vi "Actor Core.vi"(8 "error in":errorcluster, 11 "SpectrumAnalyzerUI in":refnum<class "SpectrumAnalyzerUI.lvclass">) -> (0 "error out":errorcluster, 3 "Actor out":refnum<class "Actor.lvclass">)   [LabVIEW 2023, in "SpectrumAnalyzerUI.lvlib" / "SpectrumAnalyzerUI.lvclass"]
doc: "(<B>Filename</B>: Actor Framework.lvlib:Actor.lvclass:Actor Core.vi)\n\nReceives messages to the actor, reacts to them, and initiates any error handling that may shut the actor down.\n\nDescendant classes may override this VI to append parallel tasks for the actor to complete while it handles messages. Overrides use the Call Parent Class Method node."
uses:
  SpectrumAnalyzerUI.lvclass
  <vilib>/ActorFramework/Actor/Actor.lvclass
  <vilib>/ActorFramework/Message Enqueuer/Message Enqueuer.lvclass
  Measurement_Type.ctl
  ConcreteClasses/ConcreteInstrumentClasses/KeysightN9020B/KeysightN9020B.lvclass
  <vilib>/ActorFramework/Actor/Actor.lvclass/Actor.ctl
  <vilib>/ActorFramework/Message Enqueuer/Message Enqueuer.lvclass/Message Enqueuer.ctl
  SpectrumAnalyzerUI.lvclass/SpectrumAnalyzerUI.ctl
  Interfaces/AbstractInstrumentClasses/SpectrumAnalyzer_LV/SpectrumAnalyzer Messages/ConfigureSpectrum Msg/ConfigureSpectrum Msg.lvclass/ConfigureSpectrum Msg.ctl
  Interfaces/AbstractInstrumentClasses/SpectrumAnalyzer_LV/SpectrumAnalyzer Messages/SetAverages Msg/SetAverages Msg.lvclass/SetAverages Msg.ctl
  Interfaces/InitDeinitInterface/InitDeinit Messages/Init Msg/Init Msg.lvclass/Init Msg.ctl
  Interfaces/AbstractInstrumentClasses/SpectrumAnalyzer_LV/SpectrumAnalyzer Messages/SetTrigger Msg/SetTrigger Msg.lvclass/SetTrigger Msg.ctl
  Interfaces/AbstractInstrumentClasses/SpectrumAnalyzer_LV/SpectrumAnalyzer Messages/SetAmplitudeRange Msg/SetAmplitudeRange Msg.lvclass/SetAmplitudeRange Msg.ctl
  <vilib>/ActorFramework/Message Enqueuer/Init from Existing Queue.vi
  <vilib>/ActorFramework/Message Enqueuer/Enqueue.vi
  Interfaces/AbstractInstrumentClasses/SpectrumAnalyzer_LV/SpectrumAnalyzer Messages/GetSpectrum Msg/GetSpectrum Msg.lvclass
  Interfaces/AbstractInstrumentClasses/SpectrumAnalyzer_LV/SpectrumAnalyzer Messages/ConfigureSpectrum Msg/ConfigureSpectrum Msg.lvclass
  Interfaces/AbstractInstrumentClasses/SpectrumAnalyzer_LV/SpectrumAnalyzer Messages/SetAverages Msg/SetAverages Msg.lvclass
  Interfaces/InitDeinitInterface/InitDeinit Messages/DeInit Msg/DeInit Msg.lvclass
  Interfaces/InitDeinitInterface/InitDeinit Messages/Init Msg/Init Msg.lvclass
  Interfaces/AbstractInstrumentClasses/SpectrumAnalyzer_LV/SpectrumAnalyzer Messages/SetTrigger Msg/SetTrigger Msg.lvclass
  Interfaces/AbstractInstrumentClasses/SpectrumAnalyzer_LV/SpectrumAnalyzer Messages/SetAmplitudeRange Msg/SetAmplitudeRange Msg.lvclass
  <vilib>/ActorFramework/Stop Msg/Stop Msg.lvclass
  <vilib>/ActorFramework/Message Priority Queue/Priority Enqueue.vi
  ConcreteClasses/ConcreteInstrumentClasses/KeysightN9020B/KeysightN9020B.lvlib
panel:
  out "output cluster":cluster{"Frequency":dbl[], "Amplitude":dbl[]}(graph)
  out "S-Meas Norm":dbl[][](graph)
  out "N-Meas":dbl[][](graph)
  out "S-Meas":dbl[][](graph)
  out "E-Meas":dbl[][](graph)
  out "appended array":dbl[][](graph)
  out "Measuring":bool=TRUE
  in  "attenuation":dbl caption="attenuation (dB)" min=0.0 max=10.0 step=0.1
  in  "reference level offset":dbl
  in  "reference level":dbl
  in  "Resolution BW":dbl=520.0 caption="Resolution BW (MHz)"
  in  "center frequency":dbl=520.0 caption="Center Frequency (MHz)"
  in  "span":dbl=1000.0 caption="Frequency span (MHz)"
  in  "Base Name":string="test"
  in  "file (use dialog)":path=path "D:/test"
  in  "S measurement":bool
  in  "N measurement":bool
  in  "E measurement":bool
  in  "Source":i32(ring)=1 items=["External"=1, "Immediate"=2, "Software"=3, "AC Line"=4, "Video"=5]
  in  "Trigger On":bool
  in  "ExternalTriggerLevel":dbl=1.0 caption="Trigger Level"
  out "Exiting":bool=TRUE
  out "Connected":bool
  in  "Connect":bool
  out "Measurement Type":T1=enum."S-Meas"
  out "N9020B Enqueuer":refnum<class "Message Enqueuer.lvclass">
  in  "VISA resource name":refnum<visa-resource-name>
  in  "instrument handle":refnum<k15>="N9020B"
  in  "Averages":i32
  in  "Show Spectrum":bool
  out "Self Enqueuer":refnum<class "Message Enqueuer.lvclass">
  in  "Stop Button":bool
  in  "Normalization":enum32{"(S-N)/(N-E)", "(S-E)/(E)"}(radio)=enum."(S-E)/(E)"
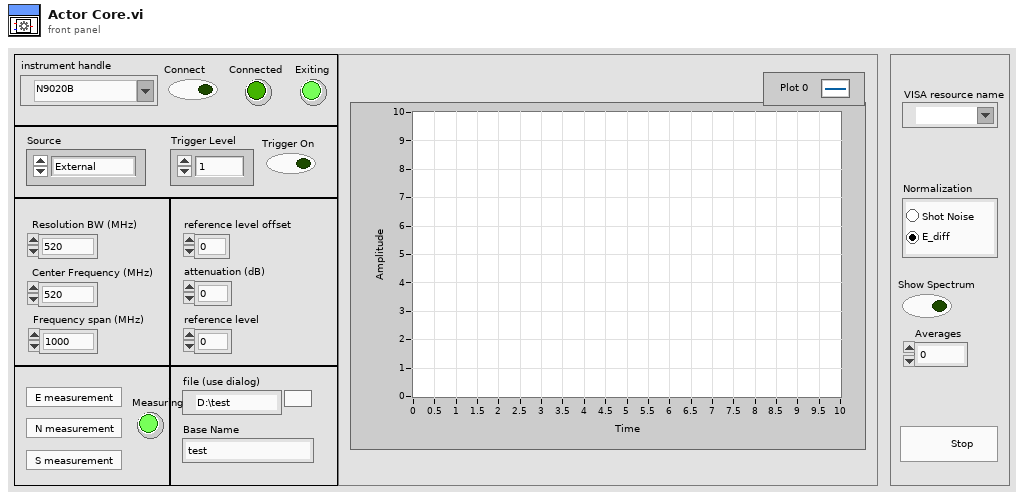
[diagram p1: front panel]
types:
  T1 = typedef "KeysightN9020B.lvlib/Measurement_Type.ctl" = enum16{"N-Meas", "S-Meas", "E-Meas", "Av_S vs Power"}
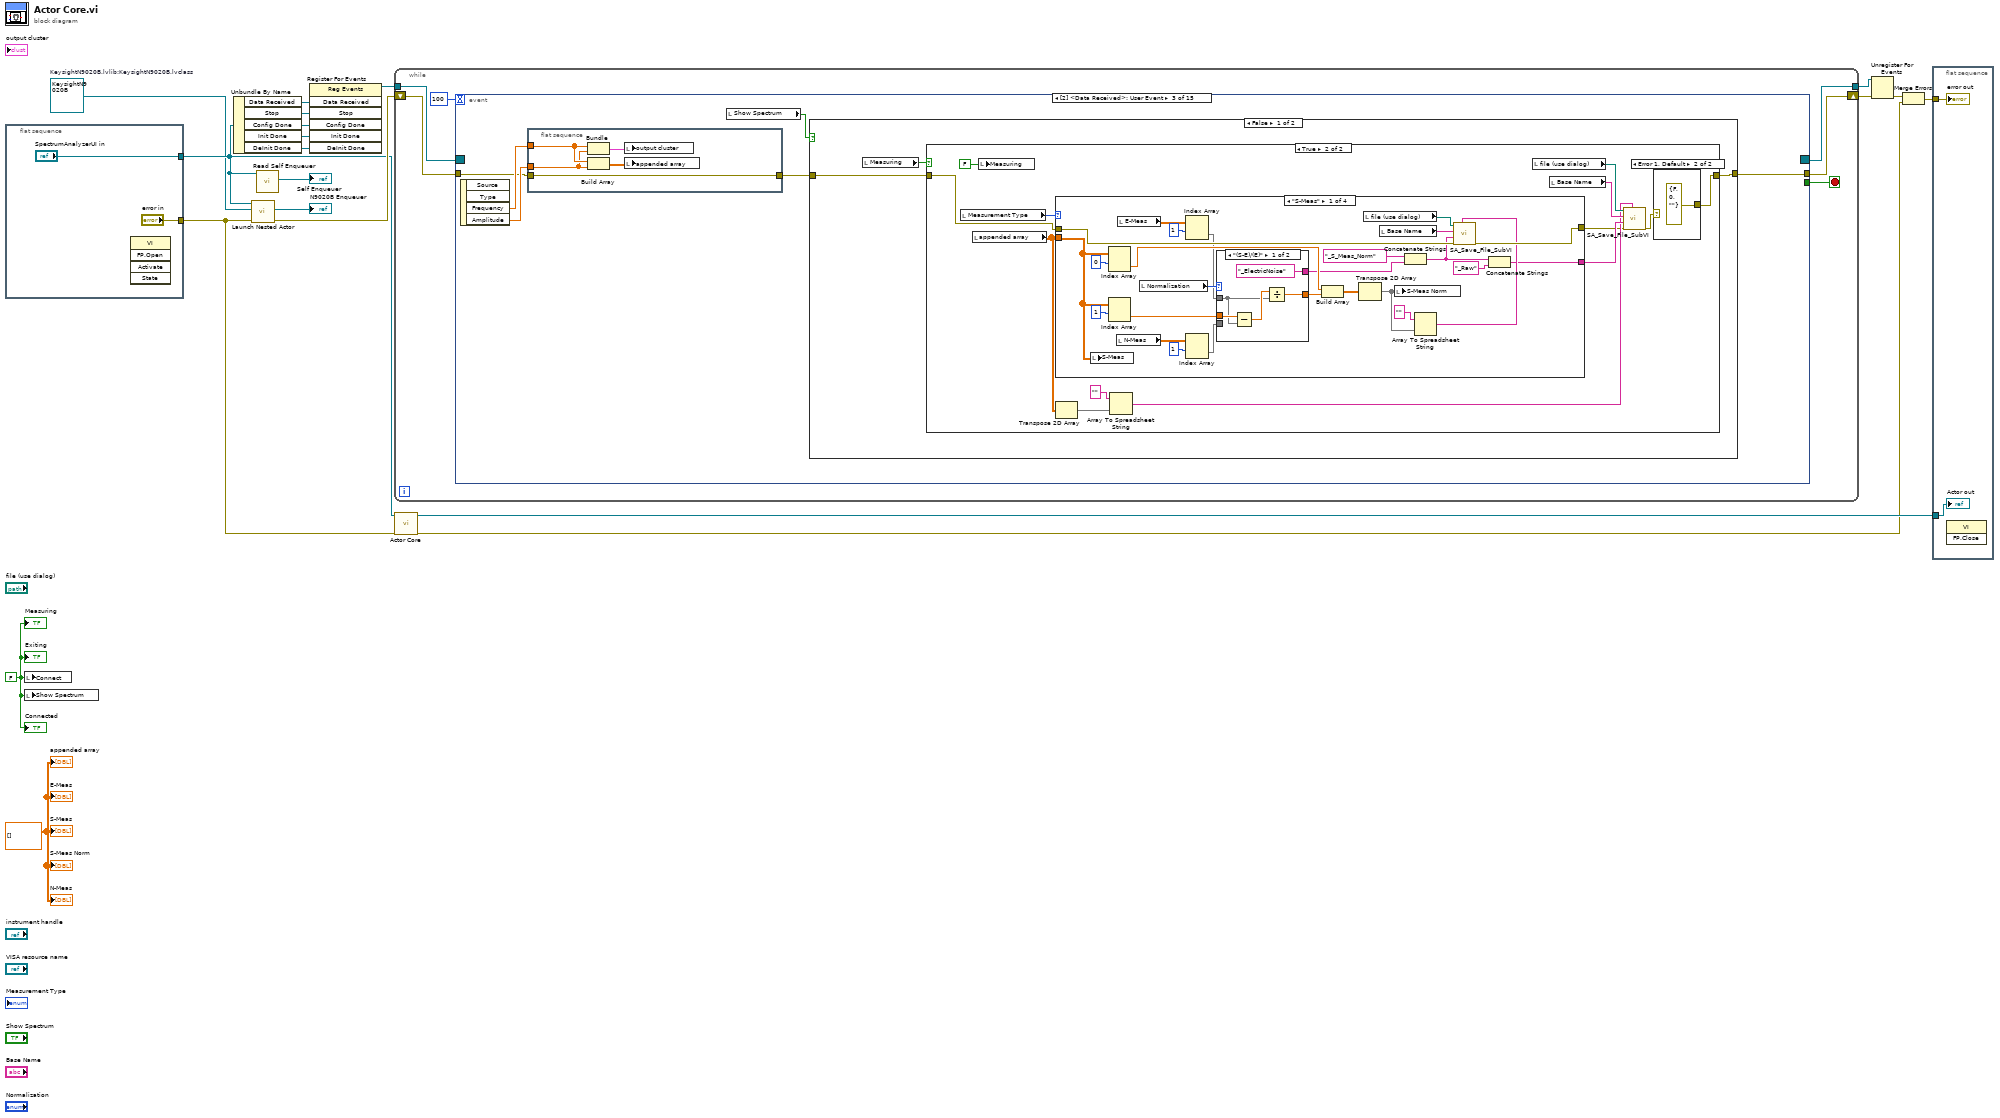
[diagram p0: block diagram]
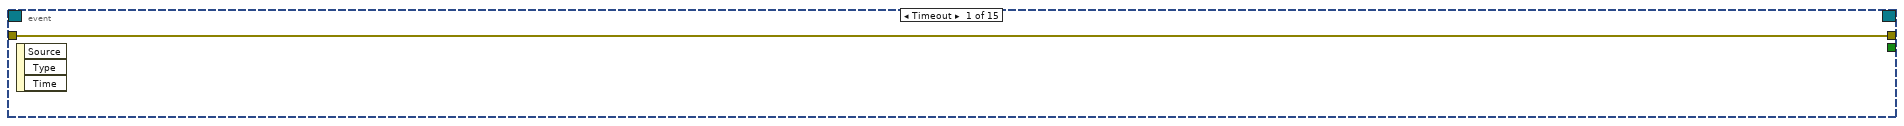
[diagram p2: hidden frame]
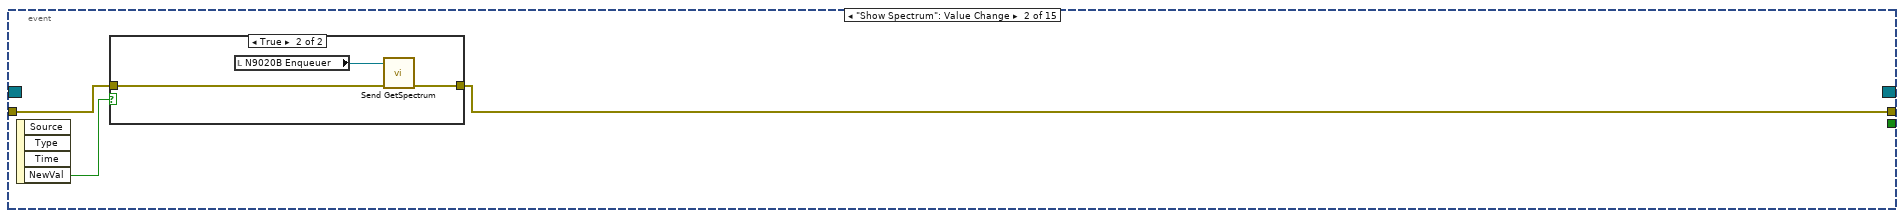
[diagram p3: hidden frame]
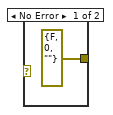
[diagram p6: hidden frame]
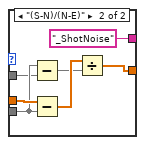
[diagram p7: hidden frame]
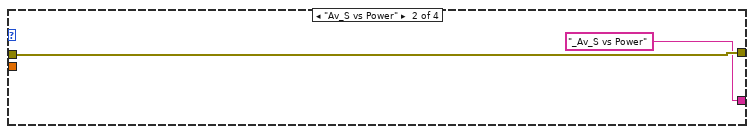
[diagram p8: hidden frame]
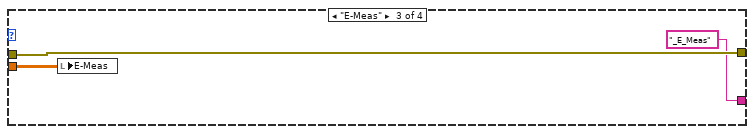
[diagram p9: hidden frame]
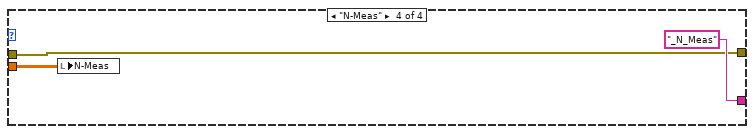
[diagram p10: hidden frame]
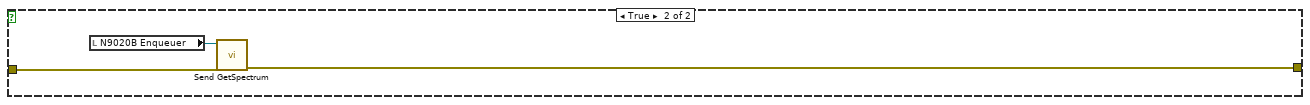
[diagram p11: hidden frame]
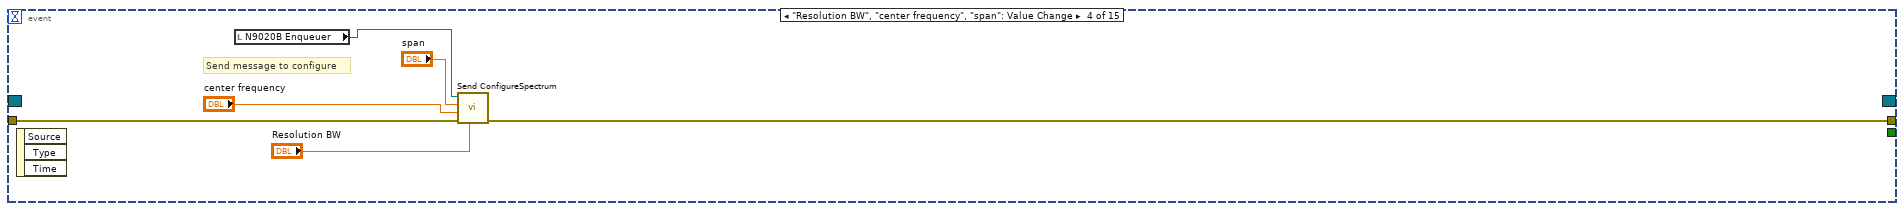
[diagram p12: hidden frame]
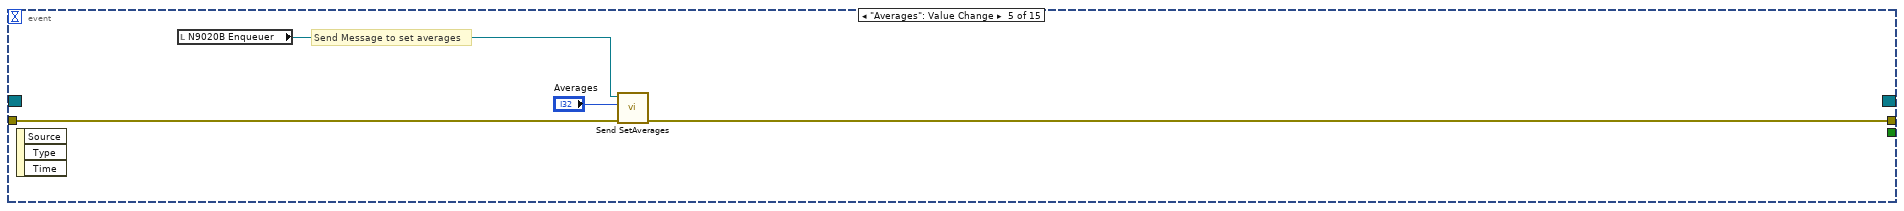
[diagram p13: hidden frame]
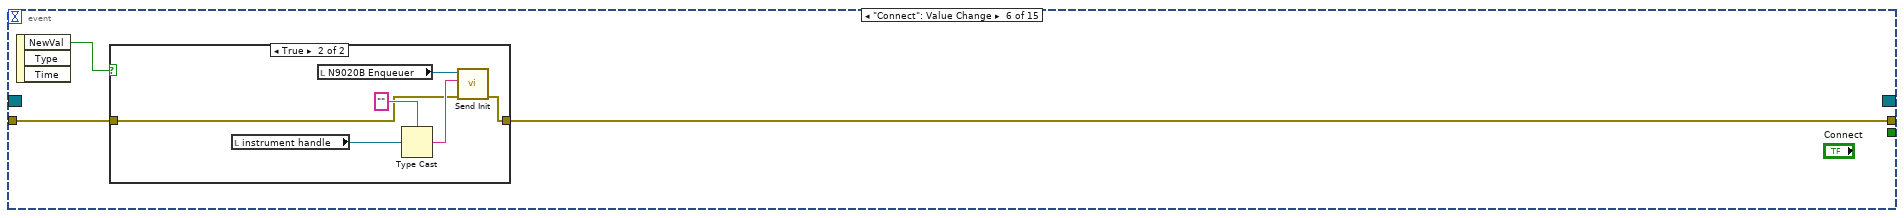
[diagram p14: hidden frame]
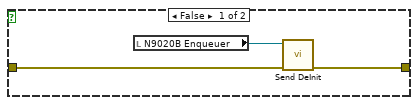
[diagram p15: hidden frame]
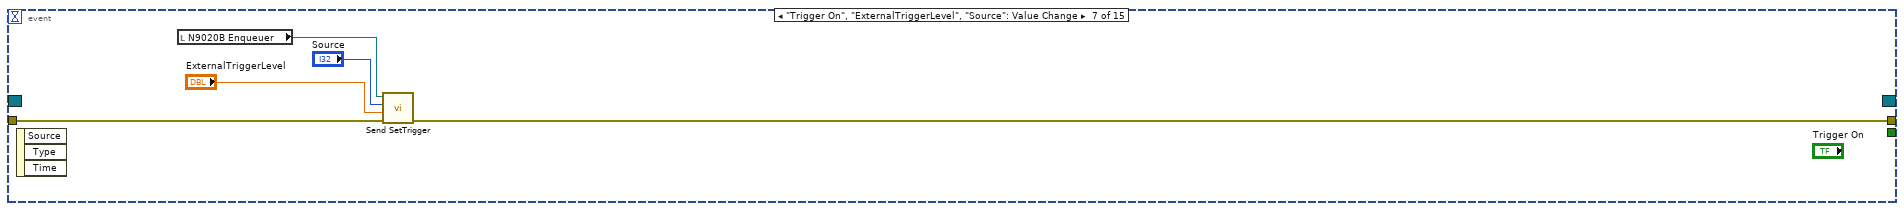
[diagram p16: hidden frame]
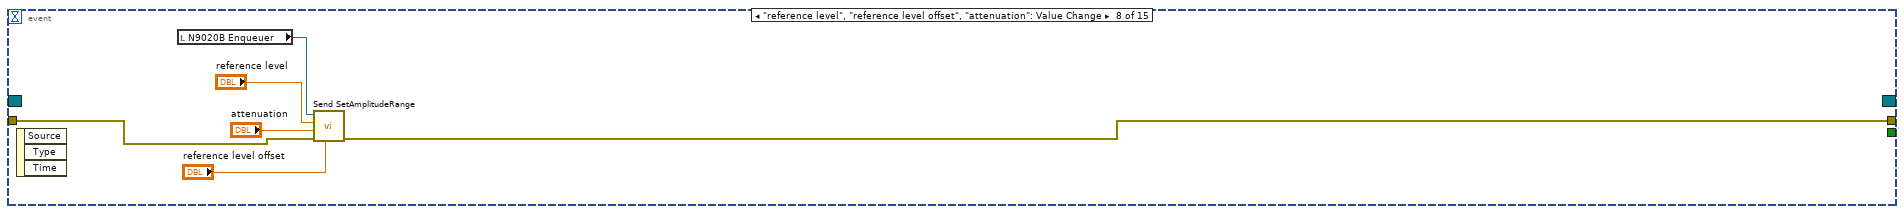
[diagram p17: hidden frame]
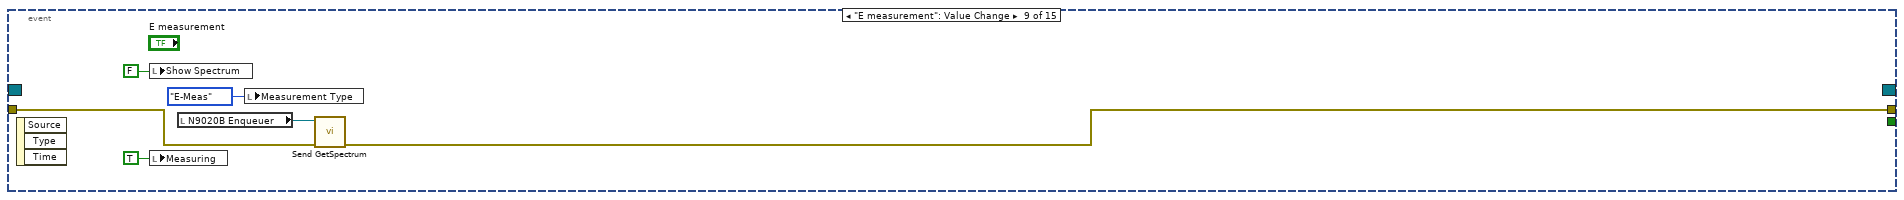
[diagram p18: hidden frame]
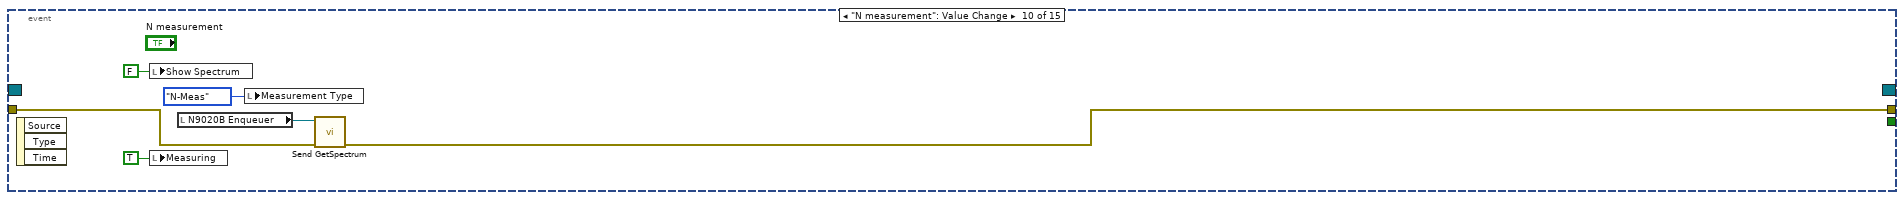
[diagram p19: hidden frame]
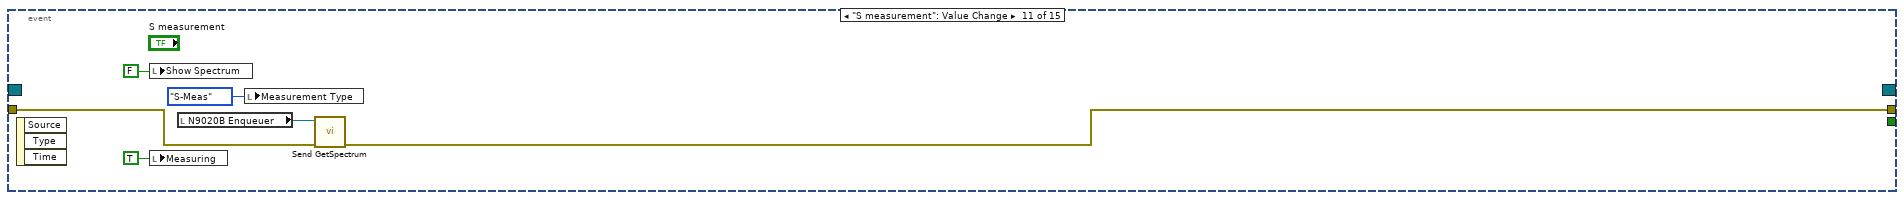
[diagram p20: hidden frame]
diagram:
  w1 = dbl[][] [] ("appended array")
  w3 = refnum<class "KeysightN9020B.lvclass"> refnum  # KeysightN9020B.lvlib:KeysightN9020B.lvclass
  w2 = FALSE ("Connected")
  n1 = flat-sequence {
    tunnel: ["error in"] -> w18
    tunnel: ["SpectrumAnalyzerUI in"] -> w15
    frame #0 {
      n2 = invoke class="VI" method="FP.Open"() -> ()  [unwired: 5 in, 5 out]
    }
  }
  n3 = local write "Connect"(w2) -> ()
  n4 = local write "Show Spectrum"(w2) -> ()
  n5 = Unbundle By Name(w15) -> ("Data Received"=w14:refnum<user-event>, "Stop"=w13:refnum<user-event>, "Config Done"=w12:refnum<user-event>, "Init Done"=w11:refnum<user-event>, "DeInit Done"=w9:refnum<user-event>)
  n6 = call <vilib>:"Launch Nested Actor.vi"("error in (no error)"=w18, "Nested Actor"=w3, "Caller Actor in"=w15) -> ("error out"=w16:errorcluster, "Nested Actor's Enqueuer"=→"N9020B Enqueuer":refnum<class "Message Enqueuer.lvclass">)  [unwired: 6 in, 1 out]
  n7 = call <vilib>:"Read Self Enqueuer.vi"("Actor"=w15) -> ("Self Enqueuer"=→"Self Enqueuer":refnum<class "Message Enqueuer.lvclass">)  [unwired: 10 in]
  n8 = register-events(w14, w13, w12, w11, w9) -> (reference out=w10:refnum<event-registration>)  [unwired: 2 in, 1 out]
  n9 = while {
    shift-right: [w27] -> w8
    shift-left: w16 -> [w28]
    tunnel: w10 -> [w25]
    tunnel: [w23] -> w4
    stop <- w24 stop-if-true
    n10 = event shown="[2] <Data Received>: User Event" {
      selector: w25 -> [_ _ _ _ _ _ _ _ _ _ _ _ _ _ _]
      dyn-events: [_ _ _ _ _ _ _ _ _ _ _ _ _ _ _] -> w23
      timeout: 100 -> [_ _ _ _ _ _ _ _ _ _ _ _ _ _ _]
      tunnel: w28 -> [w29 w31 w38 w117 w123 w128 w140 w147 w152 w158 w162 w170 w178 w182 w190]
      tunnel: [w29 w32 w41 w116 w122 w127 w139 w146 w151 w157 w161 w169 w178 w181 w190] -> w27
      tunnel: [_ _ _ _ _ _ _ _ _ _ _ _ _ _ TRUE] -> w24
      event Timeout {
        n11 = event-data() -> ()  [unwired: 1 in, 3 out]
      }
      event "Show Spectrum": Value Change {
        n12 = event-data() -> ("NewVal"=w30:bool)  [unwired: 1 in, 3 out]
        n13 = case shown="True" w30 {
          tunnel: w31 -> [w33 w35]
          tunnel: [w33 w34] -> w32
          frame False {
          }
          frame True {
            n14 = local read "N9020B Enqueuer"() -> (w36:refnum<class "Message Enqueuer.lvclass">)
            n15 = call "Send GetSpectrum.vi"("error in (no error)"=w35, "Message Enqueuer"=w36) -> ("error out"=w34:errorcluster)  [unwired: 8 in, 1 out]
          }
        }
      }
      event User Event {
        n16 = event-data() -> ("Frequency"=w40:dbl[], "Amplitude"=w39:dbl[])  [unwired: 1 in, 2 out]
        n17 = flat-sequence {
          tunnel: w40 -> [w45]
          tunnel: w39 -> [w44]
          tunnel: [w47] -> w37
          tunnel: w38 -> [w47]
          frame #0 {
            n18 = Bundle("Frequency"=w45, "Amplitude"=w44) -> (w46:cluster{"Frequency":dbl[], "Amplitude":dbl[]})  [unwired: 1 in]
            n19 = Build Array(w45, w44) -> (w43:dbl[][])
            n20 = local write "output cluster"(w46) -> ()
            n21 = local write "appended array"(w43) -> ()
          }
        }
        n22 = local read "Show Spectrum"() -> (w42:bool)
        n23 = case shown="False" w42 {
          tunnel: w37 -> [w48 w114]
          tunnel: [w49 w113] -> w41
          frame False {
            n24 = local read "Measuring"() -> (w50:bool)
            n25 = case shown="True" w50 {
              tunnel: [w51 w53] -> w49
              tunnel: w48 -> [w51 w63]
              frame False {
              }
              frame True {
                n26 = local read "Measurement Type"() -> (w64:T1)
                n27 = local read "appended array"() -> (w56:dbl[][])
                n28 = local write "Measuring"(FALSE ("Measuring")) -> ()
                n29 = case shown="\"S-Meas\"" w64 {
                  tunnel: [w88 w106 w109 w111] -> w52
                  tunnel: w63 -> [w89 w106 w109 w111]
                  tunnel: [w67 "_Av_S vs Power" ("string") "_E_Meas" ("string") "_N_Meas" ("string")] -> w59
                  tunnel: w56 -> [w79 _ w107 w110]
                  frame "S-Meas" {
                    n30 = local write "S-Meas"(w79) -> ()
                    n31 = Index Array(array=w79, index (row)=0) -> (element=w78:dbl[])  [unwired: 1 in]
                    n32 = Index Array(array=w79, index (row)=1) -> (element=w81:dbl[])  [unwired: 1 in]
                    n33 = local read "N-Meas"() -> (w83:dbl[][])
                    n34 = local read "E-Meas"() -> (w73:dbl[][])
                    n35 = local read "Normalization"() -> (w92:enum32{"(S-N)/(N-E)", "(S-E)/(E)"})
                    n36 = Index Array(array=w73, index (row)=1) -> (element=w72:dbl[])  [unwired: 1 in]
                    n37 = Index Array(array=w83, index (row)=1) -> (element=w82:dbl[])  [unwired: 1 in]
                    n38 = case shown="\"(S-E)/(E)\"" w92 {
                      tunnel: w72 -> [w95 w99]
                      tunnel: w81 -> [w97 w104]
                      tunnel: [w94 w102] -> w77
                      tunnel: w82 -> [_ w100]
                      tunnel: ["_ElectricNoise" ("string") "_ShotNoise" ("string")] -> w70
                      frame "(S-E)/(E)" {
                        n39 = Subtract(x=w97, y=w95) -> (x-y=w96:dbl[])
                        n40 = Divide(x=w96, y=w95) -> (x/y=w94:dbl[])
                      }
                      frame "(S-N)/(N-E)" {
                        n41 = Subtract(x=w100, y=w99) -> (x-y=w101:dbl[])
                        n42 = Subtract(x=w104, y=w100) -> (x-y=w103:dbl[])
                        n43 = Divide(x=w103, y=w101) -> (x/y=w102:dbl[])
                      }
                    }
                    n44 = Build Array(w78, w77) -> (w76:dbl[][])
                    n45 = Transpose 2D Array(2D array=w76) -> (transposed array=w75:dbl[][])
                    n46 = local read "file (use dialog)"() -> (w91:path)
                    n47 = local read "Base Name"() -> (w90:string)
                    n48 = local write "S-Meas Norm"(w75) -> ()
                    n49 = Concatenate Strings("_S_Meas_Norm" ("string"), w70) -> (w69:string)
                    n50 = Array To Spreadsheet String(array=w75, 3:"" ("format string")) -> (spreadsheet string=w86:string)  [unwired: 1 in]
                    n51 = call "SA_Save_File_SubVI.vi"("spreadsheet string"=w86, "error in (no error)"=w89, "string"=w69, "Base Name"=w90, "file (use dialog)"=w91) -> ("error out"=w88:errorcluster)  [unwired: 6 in]
                    n52 = Concatenate Strings(w69, "_Raw" ("string")) -> (w67:string)
                  }
                  frame "Av_S vs Power" {
                  }
                  frame "E-Meas" {
                    n53 = local write "E-Meas"(w107) -> ()
                  }
                  frame "N-Meas" {
                    n54 = local write "N-Meas"(w110) -> ()
                  }
                }
                n55 = Transpose 2D Array(2D array=w56) -> (transposed array=w55:dbl[][])
                n56 = Array To Spreadsheet String(array=w55, 3:"" ("format string")) -> (spreadsheet string=w58:string)  [unwired: 1 in]
                n57 = local read "file (use dialog)"() -> (w61:path)
                n58 = local read "Base Name"() -> (w60:string)
                n59 = call "SA_Save_File_SubVI.vi"("spreadsheet string"=w58, "error in (no error)"=w52, "string"=w59, "Base Name"=w60, "file (use dialog)"=w61) -> ("error out"=w54:errorcluster)  [unwired: 6 in]
                n60 = case shown="Error 1, Default" w54 {
                  tunnel: [errorcluster {"status"=FALSE, "code"=0, "source"=""} ("error out") errorcluster {"status"=FALSE, "code"=0, "source"=""} ("error out")] -> w53
                  frame No Error {
                  }
                  frame Error, Default {
                  }
                }
              }
            }
          }
          frame True {
            n61 = local read "N9020B Enqueuer"() -> (w115:refnum<class "Message Enqueuer.lvclass">)
            n62 = call "Send GetSpectrum.vi"("error in (no error)"=w114, "Message Enqueuer"=w115) -> ("error out"=w113:errorcluster)  [unwired: 8 in, 1 out]
          }
        }
      }
      event "Resolution BW", "center frequency", "span": Value Change {
        # "Send message to configure"
        n63 = event-data() -> ()  [unwired: 1 in, 3 out]
        n64 = local read "N9020B Enqueuer"() -> (w118:refnum<class "Message Enqueuer.lvclass">)
        n65 = call "Send ConfigureSpectrum.vi"("Resolution BW"="Resolution BW", "error in (no error)"=w117, "center frequency"="center frequency", "span"="span", "Message Enqueuer"=w118) -> ("error out"=w116:errorcluster)  [unwired: 5 in, 1 out]
      }
      event "Averages": Value Change {
        # "Send Message to set averages"
        n66 = event-data() -> ()  [unwired: 1 in, 3 out]
        n67 = local read "N9020B Enqueuer"() -> (w124:refnum<class "Message Enqueuer.lvclass">)
        n68 = call "Send SetAverages.vi"("error in (no error)"=w123, "Averages"="Averages", "Message Enqueuer"=w124) -> ("error out"=w122:errorcluster)  [unwired: 7 in, 1 out]
      }
      event "Connect": Value Change {
        n69 = event-data() -> ("NewVal"=w126:bool)  [unwired: 1 in, 2 out]
        n70 = case shown="True" w126 {
          tunnel: w128 -> [w130 w133]
          tunnel: [w129 w132] -> w127
          frame False {
            n71 = local read "N9020B Enqueuer"() -> (w131:refnum<class "Message Enqueuer.lvclass">)
            n72 = call "Send DeInit.vi"("error in (no error)"=w130, "Message Enqueuer"=w131) -> ("error out"=w129:errorcluster)  [unwired: 8 in, 1 out]
          }
          frame True {
            n73 = local read "instrument handle"() -> (w137:refnum<k15>)
            n74 = local read "N9020B Enqueuer"() -> (w134:refnum<class "Message Enqueuer.lvclass">)
            n75 = Type Cast(type="", x=w137) -> (*(type *) &x=w135:string)
            n76 = call "Send Init.vi"("error in (no error)"=w133, "Address"=w135, "Message Enqueuer"=w134) -> ("error out"=w132:errorcluster)  [unwired: 7 in, 1 out]
          }
        }
      }
      event "Trigger On", "ExternalTriggerLevel", "Source": Value Change {
        n77 = event-data() -> ()  [unwired: 1 in, 3 out]
        n78 = local read "N9020B Enqueuer"() -> (w141:refnum<class "Message Enqueuer.lvclass">)
        n79 = call "Send SetTrigger.vi"("error in (no error)"=w140, "Level"="ExternalTriggerLevel", "trigger source (External)"="Source", "Message Enqueuer"=w141) -> ("error out"=w139:errorcluster)  [unwired: 6 in, 1 out]
      }
      event "reference level", "reference level offset", "attenuation": Value Change {
        n80 = event-data() -> ()  [unwired: 1 in, 3 out]
        n81 = local read "N9020B Enqueuer"() -> (w148:refnum<class "Message Enqueuer.lvclass">)
        n82 = call "Send SetAmplitudeRange.vi"("reference level offset"="reference level offset", "error in (no error)"=w147, "Attenuation"="attenuation", "Ref Level"="reference level", "Message Enqueuer"=w148) -> ("error out"=w146:errorcluster)  [unwired: 5 in, 1 out]
      }
      event "E measurement": Value Change {
        n83 = event-data() -> ()  [unwired: 1 in, 3 out]
        n84 = local write "Show Spectrum"(FALSE ("Show Spectrum")) -> ()
        n85 = local write "Measuring"(TRUE ("Measuring")) -> ()
        n86 = local read "N9020B Enqueuer"() -> (w153:refnum<class "Message Enqueuer.lvclass">)
        n87 = local write "Measurement Type"(Measurement_Type."E-Meas" ("Measurement Type")) -> ()
        n88 = call "Send GetSpectrum.vi"("error in (no error)"=w152, "Message Enqueuer"=w153) -> ("error out"=w151:errorcluster)  [unwired: 8 in, 1 out]
      }
      event "N measurement": Value Change {
        n89 = event-data() -> ()  [unwired: 1 in, 3 out]
        n90 = local write "Show Spectrum"(FALSE ("Show Spectrum")) -> ()
        n91 = local write "Measuring"(TRUE ("Measuring")) -> ()
        n92 = local read "N9020B Enqueuer"() -> (w159:refnum<class "Message Enqueuer.lvclass">)
        n93 = local write "Measurement Type"(Measurement_Type."N-Meas" ("Measurement Type")) -> ()
        n94 = call "Send GetSpectrum.vi"("error in (no error)"=w158, "Message Enqueuer"=w159) -> ("error out"=w157:errorcluster)  [unwired: 8 in, 1 out]
      }
      event "S measurement": Value Change {
        n95 = event-data() -> ()  [unwired: 1 in, 3 out]
        n96 = local write "Show Spectrum"(FALSE ("Show Spectrum")) -> ()
        n97 = local write "Measuring"(TRUE ("Measuring")) -> ()
        n98 = local read "N9020B Enqueuer"() -> (w163:refnum<class "Message Enqueuer.lvclass">)
        n99 = local write "Measurement Type"(Measurement_Type."S-Meas" ("Measurement Type")) -> ()
        n100 = call "Send GetSpectrum.vi"("error in (no error)"=w162, "Message Enqueuer"=w163) -> ("error out"=w161:errorcluster)  [unwired: 8 in, 1 out]
      }
      event "Stop Button": Value Change {
        n101 = event-data() -> ()  [unwired: 1 in, 3 out]
        n102 = local write "Exiting"(TRUE ("Exiting")) -> ()
        n103 = local read "Connected"() -> (w167:bool)
        n104 = case shown="False" w167 {
          tunnel: w170 -> [w172 w175]
          tunnel: [w171 w174] -> w169
          frame False {
            n105 = local read "Self Enqueuer"() -> (w173:refnum<class "Message Enqueuer.lvclass">)
            n106 = call <vilib>:"Send Normal Stop.vi"("error in (no error)"=w172, "Message Enqueuer"=w173) -> ("error out"=w171:errorcluster)  [unwired: 9 in]
          }
          frame True {
            n107 = local read "N9020B Enqueuer"() -> (w176:refnum<class "Message Enqueuer.lvclass">)
            n108 = call "Send DeInit.vi"("error in (no error)"=w175, "Message Enqueuer"=w176) -> ("error out"=w174:errorcluster)  [unwired: 8 in, 1 out]
          }
        }
      }
      event User Event {
        n109 = event-data() -> ()  [unwired: 1 in, 3 out]
        n110 = local write "Connected"(TRUE ("Connected")) -> ()
      }
      event User Event {
        n111 = event-data() -> ()  [unwired: 1 in, 3 out]
        n112 = local read "Exiting"() -> (w179:bool)
        n113 = local write "Connected"(FALSE ("Connected")) -> ()
        n114 = case shown="False" w179 {
          tunnel: w182 -> [w183 w189]
          tunnel: [w183 w186] -> w181
          frame False {
          }
          frame True {
            n115 = local read "N9020B Enqueuer"() -> (w188:refnum<class "Message Enqueuer.lvclass">)
            n116 = local read "Self Enqueuer"() -> (w187:refnum<class "Message Enqueuer.lvclass">)
            n117 = call <vilib>:"Send Normal Stop.vi"("error in (no error)"=w189, "Message Enqueuer"=w188) -> ("error out"=w185:errorcluster)  [unwired: 9 in]
            n118 = call <vilib>:"Send Normal Stop.vi"("error in (no error)"=w189, "Message Enqueuer"=w187) -> ("error out"=w184:errorcluster)  [unwired: 9 in]
            n119 = Merge Errors(w185, w184) -> (w186:errorcluster)
          }
        }
      }
      event User Event {
        n120 = event-data() -> ()  [unwired: 1 in, 3 out]
      }
    }
  }
  n121 = call-parent "Actor Core.vi"("error in"=w18, "Actor in"=w15) -> ("error out"=w6:errorcluster, "Actor out"=w20:refnum<class "Actor.lvclass">)  [unwired: 8 in]
  n122 = Unregister For Events(event registration refnum=w4, error in=w8) -> (error out=w7:errorcluster)
  n123 = Merge Errors(w7, w6) -> (w5:errorcluster)
  n124 = flat-sequence {
    tunnel: w5 -> [w193]
    tunnel: w20 -> [w192]
    frame #0 {
      n125 = invoke class="VI" method="FP.Close"() -> ()  [unwired: 3 in, 3 out]
      "error out" <- w193
      "Actor out" <- w192
    }
  }
  "Connected" <- w2
  "Exiting" <- w2
  "Measuring" <- w2
  "appended array" <- w1
  "E-Meas" <- w1
  "S-Meas" <- w1
  "N-Meas" <- w1
  "S-Meas Norm" <- w1
